vi "Server_Queue Initialize.vi"(8 "error in":errorcluster) -> (0 "error out":errorcluster, 3 "Main Queue":T1)   [LabVIEW 2018, in "Cloud Server.lvlib"]
doc: "宣告伺服器程式會用到的Queue"
uses:
  Cloud Server.lvlib
  Data Def/Server_Main Queue.ctl
  Data Def/Server_Server Write Queue Data.ctl
  Data Def/Server_Main Loop Queue Data.ctl
  Data Def/Server_Main Loop State.ctl
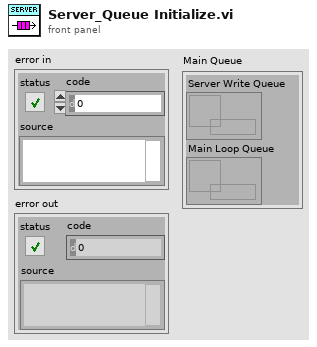
[diagram p1: front panel]
types:
  T1 = typedef "Cloud Server.lvlib/Server_Main Queue.ctl" = cluster{"Server Write Queue":refnum<queue>, "Main Loop Queue":refnum<queue>}
  T2 = typedef "Cloud Server.lvlib/Server_Main Loop Queue Data.ctl" = cluster{"Main Loop State":T3, "Data":variant}
  T3 = typedef "Cloud Server.lvlib/Server_Main Loop State.ctl" = enum16{"Detect", "Save", "Training", "Refresh User Name", "Stop"}
  T4 = typedef "Cloud Server.lvlib/Server_Server Write Queue Data.ctl" = cluster{"connection ID":refnum<k5>, "Meta Data":string, "Data":variant}
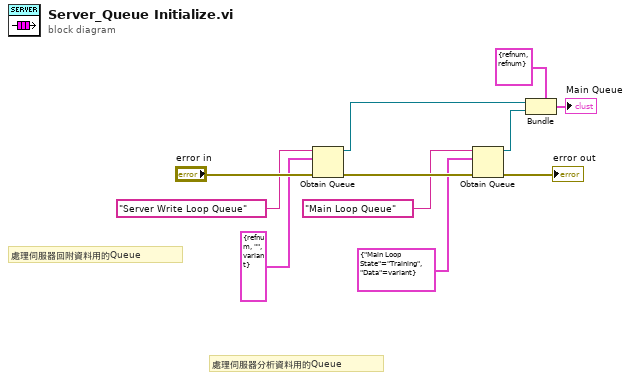
[diagram p0: block diagram]
diagram:
  # "處理伺服器分析資料用的Queue"
  # "處理伺服器回附資料用的Queue"
  n1 = Obtain Queue(name (unnamed)="Server Write Loop Queue", element data type=T4 {"connection ID"=refnum, "Meta Data"="", "Data"=variant} ("Server Write Queue Data"), error in (no error)="error in") -> (queue out=w5:refnum<queue>, error out=w8:errorcluster)  [unwired: 2 in, 1 out]
  n2 = Obtain Queue(name (unnamed)="Main Loop Queue", element data type=T2 {"Main Loop State"=enum."Training", "Data"=variant} ("Main Queue Data"), error in (no error)=w8) -> (queue out=w4:refnum<queue>, error out=→"error out":errorcluster)  [unwired: 2 in, 1 out]
  n3 = Bundle(cluster=T1 {"Server Write Queue"=refnum, "Main Loop Queue"=refnum} ("Main Queue"), "Server Write Queue"=w5, "Main Loop Queue"=w4) -> (→"Main Queue":T1)
